vi "DeletePCBModel.vi"(1 "ModelEditInfo in":T1) -> (0 "ModelEditInfo out":T1)   [LabVIEW 2014]
uses:
  <vilib>/Utility/file.llb/Write To Spreadsheet File (string).vi
  ModeEditeControl.ctl
  ModelInfo.ctl
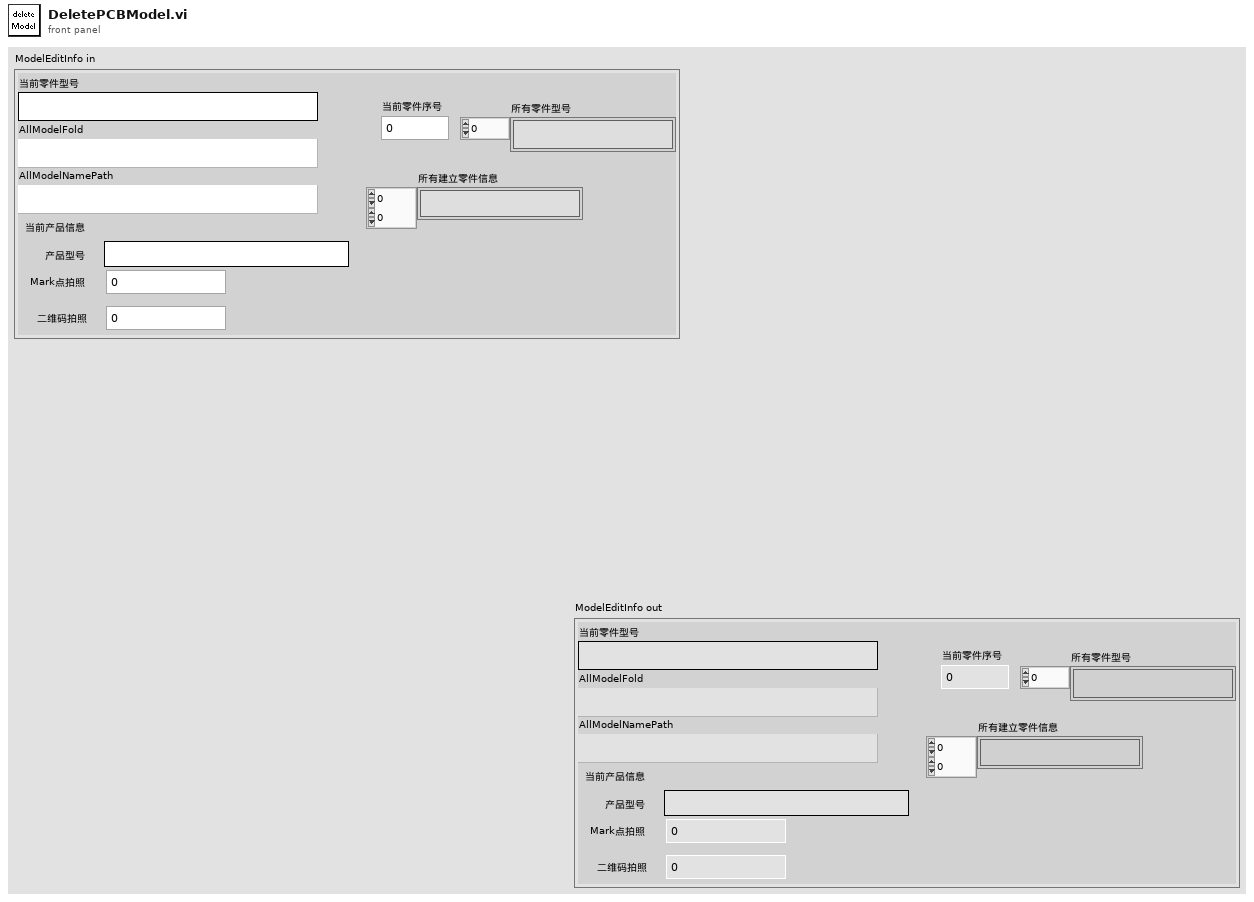
[diagram p1: front panel]
types:
  T1 = typedef "ModeEditeControl.ctl" = cluster{"AllModelFold":path, "AllModelNamePath":path, "所有零件型号":string[], "当前零件型号":string, "所有建立零件信息":string[][], "当前零件序号":i32, "当前产品信息":T2}
  T2 = typedef "ModelInfo.ctl" = cluster{"产品型号":string, "二维码拍照":u32, "Mark点拍照":u32}
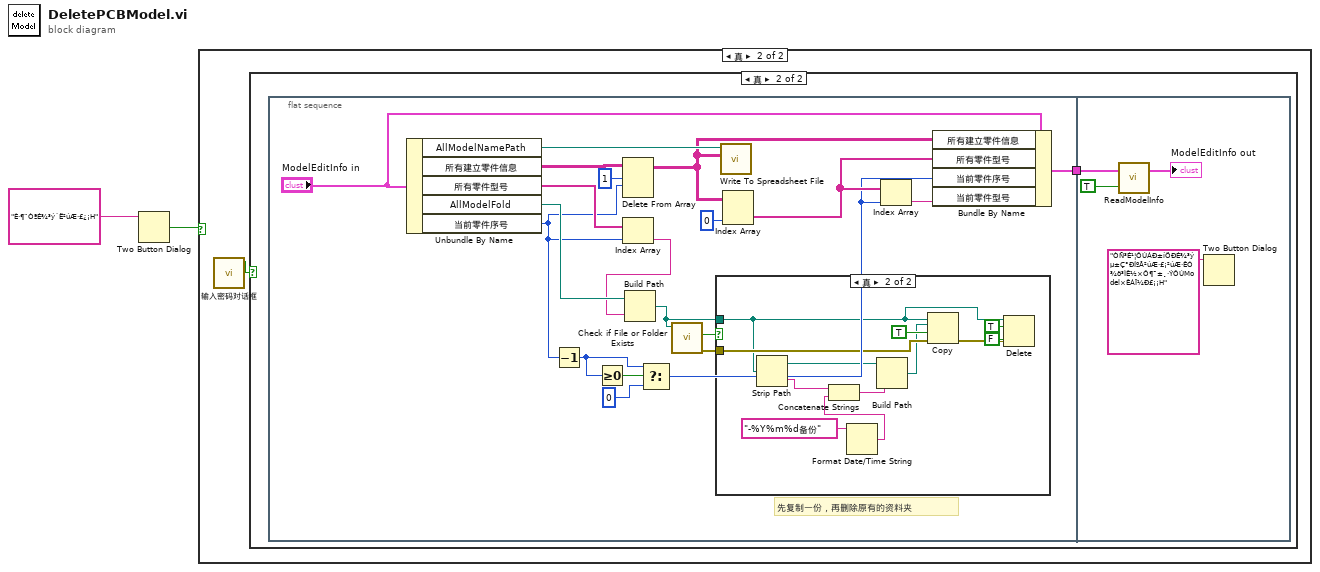
[diagram p0: block diagram]
diagram:
  n1 = Two Button Dialog(message="È·¶¨ÒªÉ¾³ý´Ë²úÆ·£¿¡H") -> (T button?=w1:bool)  [unwired: 2 in]
  n2 = case shown="真" w1 {
    frame False {
    }
    frame True {
      n3 = call "输入密码对话框.vi"() -> ("密码正确"=w3:bool)  [unwired: 11 in]
      n4 = case shown="真" w3 {
        frame False {
        }
        frame True {
          n5 = flat-sequence {
            tunnel: [w22] -> w4
            tunnel: w4 -> [w40]
            frame #0 {
              # "先复制一份，再删除原有的资料夹"
              n6 = Unbundle By Name("ModelEditInfo in") -> ("AllModelNamePath"=w24:path, "所有建立零件信息"=w19:string[][], "所有零件型号"=w10:string[], "AllModelFold"=w21:path, "当前零件序号"=w8:i32)
              n7 = Decrement(x=w8) -> (x-1=w12:i32)
              n8 = Greater Or Equal To 0?(x=w12) -> (x >= 0?=w13:bool)
              n9 = Delete From Array ("删除数组元素")(array=w19, length=1, index (row)=w8) -> (array with subset deleted=w15:string[][])  [unwired: 1 in, 1 out]
              n10 = Index Array(array=w10, index=w8) -> (element=w9:string)
              n11 = Build Path(base path=w21, name or relative path=w9) -> (appended path=w16:path)
              n12 = Select(t=w12, s=w13, f=0) -> (s? t:f=w6:i32)
              n13 = call <vilib>:"Check if File or Folder Exists.vi"("path"=w16) -> ("error out"=w17:errorcluster, "file or folder exists?"=w18:bool)  [unwired: 8 in, 1 out]
              n14 = case shown="真" w18 {
                tunnel: w16 -> [_ w31]
                tunnel: w17 -> [_ w36]
                frame False {
                }
                frame True {
                  n15 = Strip Path(path=w31) -> (stripped path=w30:path, name=w28:string)
                  n16 = Format Date/Time String(time format string (%c)="-%Y%m%d备份") -> (date/time string=w25:string)  [unwired: 2 in]
                  n17 = Concatenate Strings(w28, w25) -> (w27:string)
                  n18 = Build Path(base path=w30, name or relative path=w27) -> (appended path=w29:path)
                  n19 = Copy(8:w36, 9:TRUE ("覆盖(F)"), 10:w29, 11:w31) -> (0:w32:errorcluster)  [unwired: 1 in, 2 out]
                  n20 = Delete(path (use dialog)=w31, entire hierarchy (F)=TRUE, confirm (F)=FALSE, error in=w32) -> ()  [unwired: 1 in, 3 out]
                }
              }
              n21 = call-poly <vilib>:"Write To Spreadsheet File.vi"("2D data"=w15, "file path (dialog if empty)"=w24) -> ()  [unwired: 6 in, 1 out]
              n22 = Index Array(array=w15, index (col)=0 ("禁用的索引 (列)")) -> (element=w7:string[])  [unwired: 1 in]
              n23 = Index Array(array=w7, index=w6) -> (element=w5:string)
              n24 = Bundle By Name(cluster="ModelEditInfo in", "所有建立零件信息"=w15, "所有零件型号"=w7, "当前零件序号"=w6, "当前零件型号"=w5) -> (w22:T1)
            }
            frame #1 {
              n25 = call "ReadModelInfo.vi"("更新量测项目序号"=TRUE, "ModelEditInfo in"=w40) -> ("ModelEditInfo out"=→"ModelEditInfo out":T1)  [unwired: 1 in]
              n26 = Two Button Dialog(message="ÒÑ³É¹¦ÔÚÁÐ±íÖÐÉ¾³ýµ±Ç°ÐÍºÅ²úÆ·£¡²úÆ·ÊÓ¾õ³ÌÊ½×Ô¶¯±¸·ÝÔÚModel×ÊÁÏ¼Ð£¡¡H") -> ()  [unwired: 2 in, 1 out]
            }
          }
        }
      }
    }
  }
